vi "Write Q1 Data.vi"(9 "Q1 Data in":string[][](array[string]), 10 "section":string, 11 "CalOption":enum32{"Positive", "Negative"}(ring)) -> ()   [LabVIEW 2015]
uses:
  <vilib>/Utility/config.llb/Write Key (String).vi
  <vilib>/Utility/config.llb/NI_LVConfig.lvlib
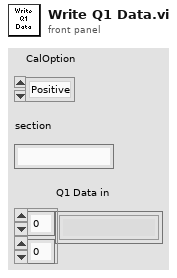
[diagram p1: front panel]
types:
  T1 = typedef "NI_LVConfig.lvlib/Config Data RefNum.ctl" = refnum<k1>
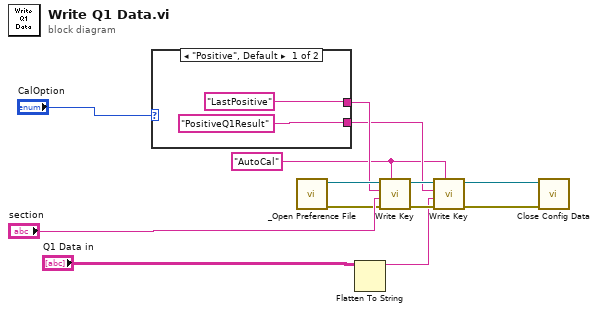
[diagram p0: block diagram]
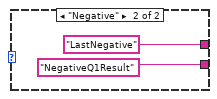
[diagram p2: hidden frame]
diagram:
  w3 = "AutoCal" ("section")
  n1 = case shown="\"Positive\", Default" "CalOption" {
    tunnel: ["LastPositive" ("section") "LastNegative" ("section")] -> w6
    tunnel: ["PositiveQ1Result" ("section") "NegativeQ1Result" ("section")] -> w5
    frame "Positive", Default {
    }
    frame "Negative" {
    }
  }
  n2 = call "_Open Preference File.vi"() -> ("error"=w8:errorcluster, "refnum"=w10:T1)  [unwired: 3 in, 3 out]
  n3 = Flatten To String(anything="Q1 Data in") -> (data string=w4:string)  [unwired: 3 in, 2 out]
  n4 = call-poly <vilib>:"Write Key.vi"("section"=w3, "error in (no error)"=w8, "value"="section", "key"=w6, "refnum"=w10) -> ("error out"=w7:errorcluster, "refnum out"=w9:T1)  [unwired: 4 in, 1 out]
  n5 = call-poly <vilib>:"Write Key.vi"("section"=w3, "error in (no error)"=w7, "value"=w4, "key"=w5, "refnum"=w9) -> ("error out"=w1:errorcluster, "refnum out"=w2:T1)  [unwired: 4 in, 1 out]
  n6 = call <vilib>:"Close Config Data.vi"("error in (no error)"=w1, "refnum"=w2) -> ()  [unwired: 1 in, 9 out]
